vi "shag_start — 8.vi"() -> ()   [LabVIEW 2016]
uses:
  <vilib>/Instr/_visa.llb/VISA Configure Serial Port (Instr).vi
panel:
  out "text":string
  out "2":i32
  out "1":i32
  out "text2":string
  out "положение в мин 2":i32
  out "положение в мин 1":i32
  in  "all":T1(tab)
  out "положение шд 2":i32(knob) scale=-10.0..190.0
  out "текущее положение 2":string
  out "положение в минутах 2":string
  in  "Минуты 2":i32 min=-600 max=11400
  in  "Stop двигатель 2":bool
  in  "Вращение по градусам +  2":bool
  in  "Вращение по градусам -  2":bool
  in  "Вернуться в нулевое положение 2":bool
  in  "Задать текущее положение нулевым 2":bool
  in  "Установка минут 2":bool
  in  "Блокировать трубку №2":bool
  out "положение шд":i32(knob) scale=-10.0..190.0
  out "текущее положение":string
  out "положение в минутах 1":string
  in  "Минуты":i32 min=-600 max=11400
  in  "Stop двигатель":bool
  in  "Вращение по градусам +":bool
  in  "Вращение по градусам -":bool
  in  "Вернуться в нулевое положение":bool
  in  "Задать текущее положение нулевым":bool
  in  "Установка минут":bool
  in  "Блокировать зеркало №1":bool
  in  "stop":bool
  in  "Выберете COM порт":refnum<visa-resource-name>="COM1"
  in  "Скорость обмена данными":u32(ring)=19200 items=["9600"=9600, "19200"=19200, "38400"=38400, "57600"=57600]
  in  "Число бит на символ":u16=8 min=5 max=8 step=1
  in  "Контроль чётности":enum16{"None", "Odd", "Even", "Mark", "Space"}(ring)
  in  "Стоповый бит":u16(ring)=10 items=["1.0"=10, "1.5"=15, "2.0"=20]
  in  "Контроль переполнения":u16(ring) items=["None"=0, "XON/XOFF"=1, "RTS/CTS"=2, "DTR/DSR"=4]
  # "1 - адресс 1 двигателя\n2 - адресс 2 двигателя\n$0MV\\01+   - запуск всех двигателей в положительном направлении \n$0MS\\00   - остановка всех двигателей\n$0MJ\\04+\\00\\00\\01   - 1 шаг всех двигателей\n$0SS\\01\\10   - скорость 10 для всех двигателей"
  # "Поворотный стол"
  # "Ренгеновская трубка №2"
  # "Положение:"
  # "Зеркало №1"
  # "Положение:"
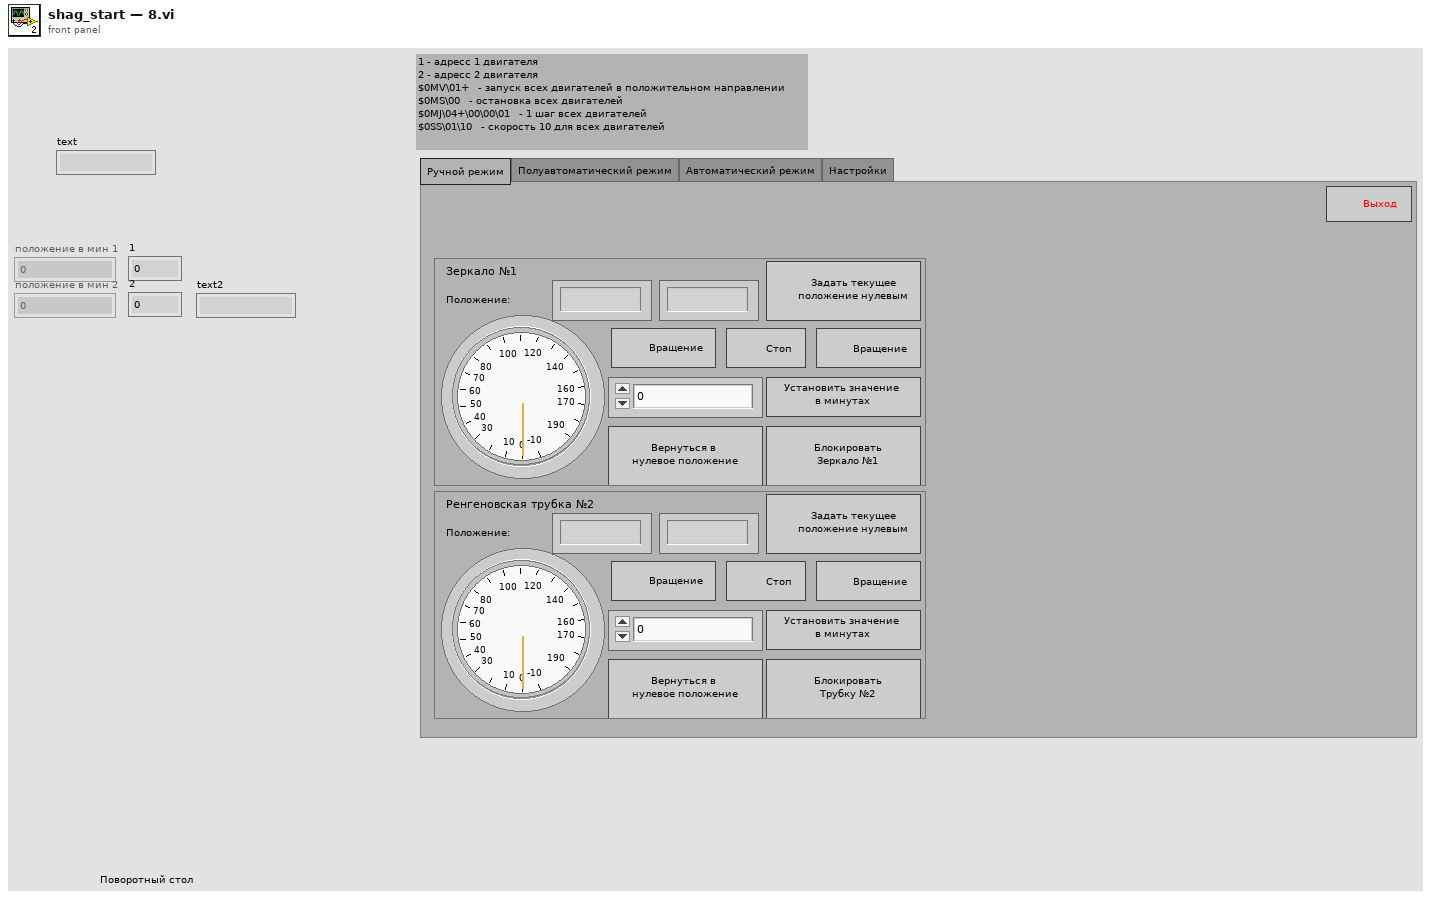
[diagram p1: front panel]
types:
  T1 = enum32{"Ручной режим", "Полуавтоматический режим", "Автоматический режим", "Настройки"}
  T2 = enum16{"open", "replace", "create", "open or create", "replace or create", "replace or create with confirmation"}
  T3 = enum8{"Enabled", "Disabled", "Disabled and Grayed Out"}
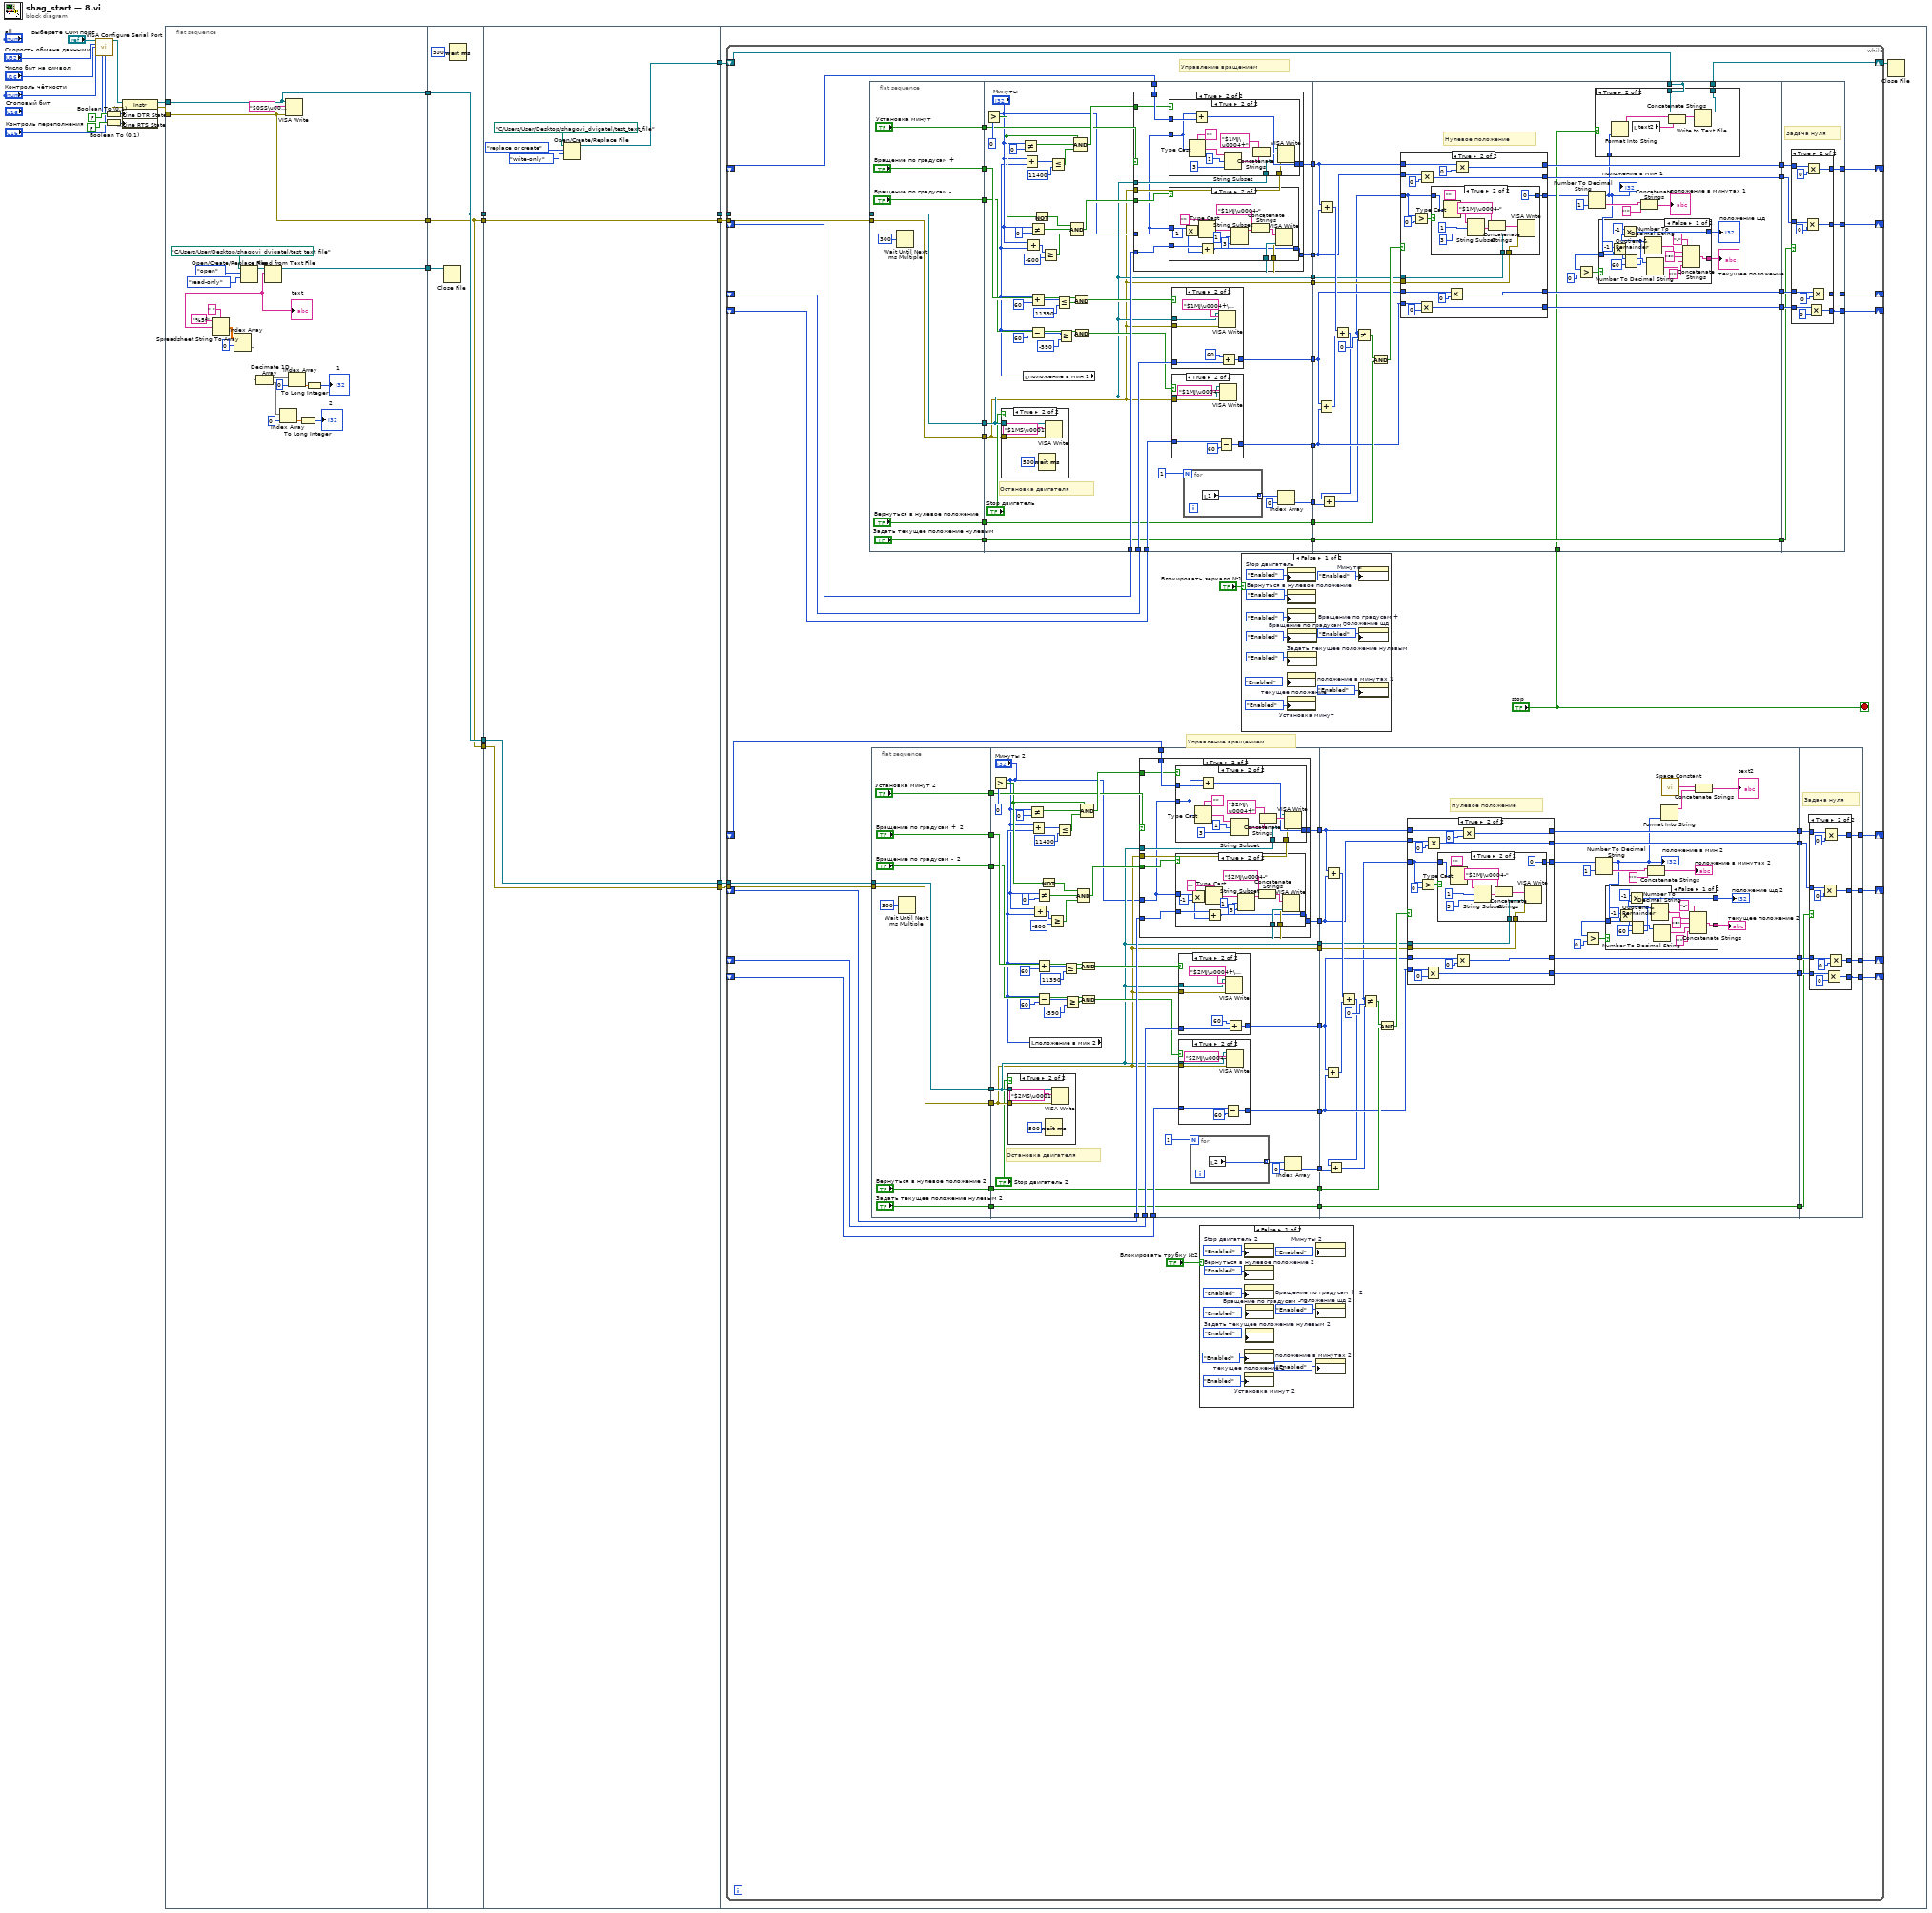
[diagram p0: block diagram]
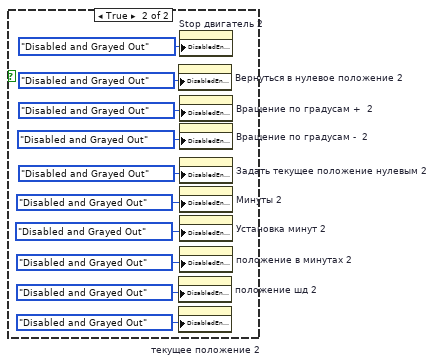
[diagram p2: hidden frame]
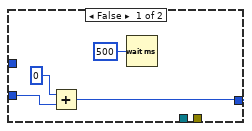
[diagram p4: hidden frame]
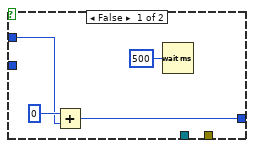
[diagram p5: hidden frame]
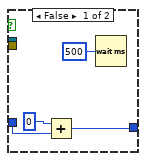
[diagram p7: hidden frame]
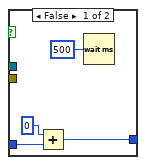
[diagram p8: hidden frame]
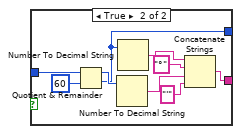
[diagram p9: hidden frame]
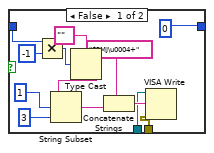
[diagram p11: hidden frame]
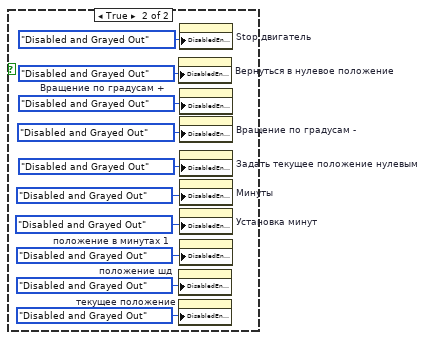
[diagram p13: hidden frame]
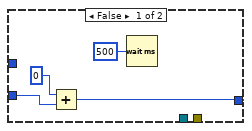
[diagram p15: hidden frame]
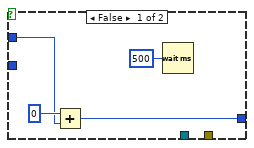
[diagram p16: hidden frame]
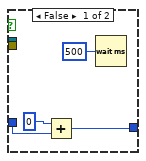
[diagram p18: hidden frame]
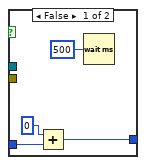
[diagram p19: hidden frame]
diagram:
  n1 = call-poly "VISA Configure Serial Port"("VISA resource name"="Выберете COM порт", "baud rate (9600)"="Скорость обмена данными", "data bits (8)"="Число бит на символ", "parity (0:none)"="Контроль чётности", "stop bits (10: 1 bit)"="Стоповый бит", "flow control (0:none)"="Контроль переполнения") -> ("VISA resource name out"=w24:refnum<visa-resource-name>, "error out"=w23:errorcluster)  [unwired: 8 in]
  n2 = Boolean To (0,1)(Boolean=FALSE ("DTR Write")) -> (0, 1=w25:i16)
  n3 = Boolean To (0,1)(Boolean=FALSE ("DTR Write")) -> (0, 1=w26:i16)
  n4 = property class="Instr"(reference=w24, error in=w23, "Serial Settings:Modem Line Settings:Line DTR State"=w25, "Serial Settings:Modem Line Settings:Line RTS State"=w26) -> (reference out=w22:refnum<visa-resource-name>, error out=w21:errorcluster)
  n5 = flat-sequence {
    tunnel: w22 -> [w47]
    tunnel: w21 -> [w46]
    tunnel: [w47] -> w20
    tunnel: [w46] -> w19
    tunnel: [w42] -> w10
    tunnel: [w51] -> w9
    tunnel: w20 -> [w51]
    tunnel: w19 -> [w50]
    tunnel: [w50] -> w7
    tunnel: [w51] -> w5
    tunnel: [w50] -> w3
    tunnel: w10 -> [w49]
    tunnel: w9 -> [w60]
    tunnel: [w60] -> w8
    tunnel: w7 -> [w59]
    tunnel: [w59] -> w6
    tunnel: w5 -> [w58]
    tunnel: [w58] -> w4
    tunnel: w3 -> [w57]
    tunnel: [w57] -> w2
    tunnel: [w53] -> w1
    tunnel: w8 -> [w66]
    tunnel: w6 -> [w65]
    tunnel: w4 -> [w61]
    tunnel: w2 -> [w64]
    tunnel: w1 -> [w63]
    frame #0 {
      n6 = Open/Create/Replace File(file path (use dialog)=path "C:/Users/User/Desktop/shagovi_dvigatel/test_text_file", operation (0:open)=T2."open", access (0:read/write)=enum16{"read/write", "read-only", "write-only"}."read-only") -> (refnum out=w41:refnum<file>)  [unwired: 3 in, 2 out]
      n7 = Read from Text File(file (use dialog)=w41) -> (refnum out=w42:refnum<file>, text=w27:string)  [unwired: 3 in, 2 out]
      "text" <- w27
      n8 = Spreadsheet String To Array(delimiter (Tab)=" ", format string="%5f", spreadsheet string=w27) -> (array=w38:dbl[][])  [unwired: 1 in]
      n9 = Index Array(array=w38, index (row)=0 ("index")) -> (element=w36:dbl[])  [unwired: 1 in]
      n10 = Decimate 1D Array(w36) -> (w32:dbl[], w34:dbl[])
      n11 = Index Array(array=w34, index=0) -> (element=w31:dbl)
      n12 = VISA Write(VISA resource name=w47, write buffer="$0SS\u0001\u0010", error in (no error)=w46) -> ()  [unwired: 3 out]
      n13 = Index Array(array=w32, index=0) -> (element=w30:dbl)
      n14 = To Long Integer(number=w31) -> (32bit integer=→"2":i32)
      n15 = To Long Integer(number=w30) -> (32bit integer=→"1":i32)
    }
    frame #1 {
      n16 = Close File(refnum=w49) -> ()  [unwired: 1 in, 2 out]
      n17 = Wait (ms)(milliseconds to wait=u32 500) -> ()  [unwired: 1 out]
    }
    frame #2 {
      n18 = Open/Create/Replace File(file path (use dialog)=path "C:/Users/User/Desktop/shagovi_dvigatel/test_text_file", operation (0:open)=T2."replace or create", access (0:read/write)=enum16{"read/write", "read-only", "write-only"}."write-only") -> (refnum out=w53:refnum<file>)  [unwired: 3 in, 2 out]
    }
    frame #3 {
      n19 = while {
        tunnel: w66 -> [w109]
        tunnel: w65 -> [w108]
        shift-right: [w104] -> _
        shift-left: _ -> [w113]
        shift-right: [w105] -> _
        shift-left: _ -> [w112]
        shift-right: [w106] -> _
        shift-left: _ -> [w111]
        shift-right: [w107] -> _
        shift-left: _ -> [w110]
        tunnel: w64 -> [w78]
        shift-right: [w100] -> w62
        shift-left: w63 -> [w101]
        tunnel: w61 -> [w77]
        shift-right: [w73] -> _
        shift-left: _ -> [w74]
        shift-right: [w71] -> _
        shift-left: _ -> [w72]
        shift-right: [w69] -> _
        shift-left: _ -> [w70]
        shift-right: [w67] -> _
        shift-left: _ -> [w68]
        stop <- "stop" stop-if-true
        # "Управление вращением"
        # "Управление вращением"
        n20 = flat-sequence {
          tunnel: w108 -> [w432]
          tunnel: w109 -> [w433]
          tunnel: [w433] -> w133
          tunnel: [w432] -> w132
          tunnel: ["Вращение по градусам +"] -> w131
          tunnel: ["Вращение по градусам -"] -> w130
          tunnel: ["Вернуться в нулевое положение"] -> w129
          tunnel: ["Задать текущее положение нулевым"] -> w128
          tunnel: ["Установка минут"] -> w127
          tunnel: w133 -> [w457]
          tunnel: w132 -> [w439]
          tunnel: [w480] -> w126
          tunnel: w113 -> [w477]
          tunnel: w112 -> [w479]
          tunnel: [w478] -> w125
          tunnel: w111 -> [w476]
          tunnel: w110 -> [w475]
          tunnel: w131 -> [w461]
          tunnel: w130 -> [w460]
          tunnel: [w474] -> w124
          tunnel: [w473] -> w123
          tunnel: [w458] -> w122
          tunnel: w129 -> [w458]
          tunnel: [w439] -> w121
          tunnel: [w457] -> w120
          tunnel: [w456] -> w119
          tunnel: w128 -> [w456]
          tunnel: w127 -> [w450]
          tunnel: [w437] -> w102
          tunnel: w126 -> [w562]
          tunnel: w125 -> [w563]
          tunnel: [w582] -> w118
          tunnel: [w580] -> w117
          tunnel: w124 -> [w564]
          tunnel: w123 -> [w565]
          tunnel: [w571] -> w116
          tunnel: [w578] -> w115
          tunnel: w122 -> [w574]
          tunnel: w121 -> [w570]
          tunnel: w120 -> [w569]
          tunnel: w119 -> [w567]
          tunnel: [w567] -> w114
          tunnel: [w556] -> _
          tunnel: "stop" -> [w559]
          tunnel: w101 -> [w556]
          tunnel: w102 -> [w551]
          tunnel: [w552] -> w100
          tunnel: [w668] -> w104
          tunnel: [w665] -> w105
          tunnel: w118 -> [w667]
          tunnel: w117 -> [w666]
          tunnel: [w664] -> w106
          tunnel: [w663] -> w107
          tunnel: w116 -> [w662]
          tunnel: w115 -> [w661]
          tunnel: w114 -> [w660]
          frame #0 {
            n21 = Wait Until Next ms Multiple(millisecond multiple=u32 300) -> ()  [unwired: 1 out]
          }
          frame #1 {
            # "Остановка двигателя"
            n22 = Greater?(x="Минуты", y=0) -> (0:w448:bool)
            n23 = case shown="True" "Stop двигатель" {
              tunnel: w457 -> [_ w528]
              tunnel: w439 -> [_ w527]
              frame False {
              }
              frame True {
                n24 = Wait (ms)(milliseconds to wait=u32 500) -> ()  [unwired: 1 out]
                n25 = VISA Write(VISA resource name=w528, write buffer="$1MS\u0001", error in (no error)=w527) -> ()  [unwired: 3 out]
              }
            }
            n26 = Not Equal?(x="Минуты", y=0) -> (x != y?=w447:bool)
            n27 = local read "положение в мин 1"() -> (w438:i32)
            n28 = Add(x="Минуты", y=w438) -> (x+y=w471:i32)
            n29 = Add(x="Минуты", y=w438) -> (x+y=w442:i32)
            n30 = Not Equal?(x="Минуты", y=0) -> (x != y?=w445:bool)
            n31 = Add(x=w438, y=60) -> (x+y=w466:i32)
            n32 = Subtract(x=w438, y=60) -> (x-y=w453:i32)
            n33 = Not(x=w448) -> (.not. x?=w449:bool)
            n34 = Greater Or Equal?(x=w442, y=-600) -> (x >= y?=w443:bool)
            n35 = Less Or Equal?(x=w471, y=11400) -> (x <= y?=w446:bool)
            n36 = Less Or Equal?(x=w466, y=11390) -> (x <= y?=w463:bool)
            n37 = Greater Or Equal?(x=w453, y=-590) -> (x >= y?=w454:bool)
            n38 = Compound Arithmetic op=AND(w449, w445, w443) -> (w467:bool)
            n39 = And(x=w461, y=w463) -> (x .and. y?=w462:bool)
            n40 = And(x=w460, y=w454) -> (x .and. y?=w459:bool)
            n41 = Compound Arithmetic op=AND(w448, w447, w446) -> (w469:bool)
            n42 = case shown="True" w450 {
              tunnel: [w483 w492] -> w480
              tunnel: w479 -> [w482 w491]
              tunnel: [w482 w490] -> w478
              tunnel: w477 -> [w483 w489]
              tunnel: w469 -> [_ w488]
              tunnel: w467 -> [_ w487]
              tunnel: w439 -> [_ w486]
              tunnel: w457 -> [_ w485]
              tunnel: "Минуты" -> [_ w484]
              frame False {
              }
              frame True {
                n43 = case shown="True" w488 {
                  tunnel: [w513 w519] -> w492
                  tunnel: w489 -> [w512 w518]
                  tunnel: w486 -> [_ w517]
                  tunnel: w485 -> [_ w516]
                  tunnel: w484 -> [_ w515]
                  frame False {
                    n44 = Add(x=0, y=w512) -> (x+y=w513:i32)
                    n45 = Wait (ms)(milliseconds to wait=u32 500) -> ()  [unwired: 1 out]
                  }
                  frame True {
                    n46 = Type Cast(type="", x=w515) -> (*(type *) &x=w522:string)
                    n47 = Add(x=w515, y=w518) -> (x+y=w519:i32)
                    n48 = String Subset(string=w522, offset (0)=1, length (rest)=3 ("length (rest)")) -> (substring=w521:string)
                    n49 = Concatenate Strings("$1MJ\u0004+" ("write buffer"), w521) -> (w525:string)
                    n50 = VISA Write(VISA resource name=w516, write buffer=w525, error in (no error)=w517) -> ()  [unwired: 3 out]
                  }
                }
                n51 = case shown="True" w487 {
                  tunnel: [w495 w501] -> w490
                  tunnel: w491 -> [w494 w500]
                  tunnel: w485 -> [_ w503]
                  tunnel: w486 -> [_ w502]
                  tunnel: w484 -> [_ w497]
                  frame False {
                    n52 = Add(x=0, y=w494) -> (x+y=w495:i32)
                    n53 = Wait (ms)(milliseconds to wait=u32 500) -> ()  [unwired: 1 out]
                  }
                  frame True {
                    n54 = Multiply(x=w497, y=-1) -> (x*y=w499:i32)
                    n55 = Type Cast(type="", x=w499) -> (*(type *) &x=w506:string)
                    n56 = Add(x=w500, y=w497) -> (x+y=w501:i32)
                    n57 = String Subset(string=w506, offset (0)=1, length (rest)=3 ("length (rest)")) -> (substring=w505:string)
                    n58 = Concatenate Strings("$1MJ\u0004-" ("write buffer"), w505) -> (w509:string)
                    n59 = VISA Write(VISA resource name=w503, write buffer=w509, error in (no error)=w502) -> ()  [unwired: 3 out]
                  }
                }
              }
            }
            n60 = case shown="True" w462 {
              tunnel: [w543 w550] -> w474
              tunnel: w476 -> [w542 w545]
              tunnel: w457 -> [_ w546]
              tunnel: w439 -> [_ w547]
              frame False {
                n61 = Add(x=0, y=w542) -> (x+y=w543:i32)
                n62 = Wait (ms)(milliseconds to wait=u32 500) -> ()  [unwired: 1 out]
              }
              frame True {
                n63 = VISA Write(VISA resource name=w546, write buffer="$1MJ\u0004+\u0000\u0000<", error in (no error)=w547) -> ()  [unwired: 3 out]
                n64 = Add(x=60, y=w545) -> (x+y=w550:i32)
              }
            }
            n65 = case shown="True" w459 {
              tunnel: [w533 w536] -> w473
              tunnel: w475 -> [w532 w535]
              tunnel: w457 -> [_ w539]
              tunnel: w439 -> [_ w538]
              frame False {
                n66 = Add(x=0, y=w532) -> (x+y=w533:i32)
                n67 = Wait (ms)(milliseconds to wait=u32 500) -> ()  [unwired: 1 out]
              }
              frame True {
                n68 = Subtract(x=w535, y=60 ("x")) -> (x-y=w536:i32)
                n69 = VISA Write(VISA resource name=w539, write buffer="$1MJ\u0004-\u0000\u0000<", error in (no error)=w538) -> ()  [unwired: 3 out]
              }
            }
            n70 = for {
              N: 1 -> [_]
              tunnel: [w481] -> w435 mode=indexing
              n71 = local read "1"() -> (w481:i32)
            }
            n72 = Index Array(array=w435, index=0) -> (element=w437:i32)
          }
          frame #2 {
            # "Нулевое положение"
            n73 = Add(x=w564, y=w565) -> (x+y=w575:i32)
            n74 = Add(x=w562, y=w563) -> (x+y=w579:i32)
            n75 = Add(x=w579, y=w575) -> (x+y=w554:i32)
            n76 = Add(x=w554, y=w551) -> (x+y=w553:i32)
            n77 = Not Equal?(x=w553, y=0 ("x")) -> (x != y?=w572:bool)
            n78 = And(x=w572, y=w574) -> (x .and. y?=w581:bool)
            n79 = case shown="True" w581 {
              tunnel: [w613 w635] -> w555
              tunnel: w562 -> [w617 w632]
              tunnel: [w617 w631] -> w582
              tunnel: [w616 w630] -> w580
              tunnel: w553 -> [w613 w624]
              tunnel: [w614 w626] -> w578
              tunnel: [w615 w623] -> w571
              tunnel: w563 -> [w616 w622]
              tunnel: w570 -> [_ w621]
              tunnel: w569 -> [_ w620]
              tunnel: w564 -> [w615 w619]
              tunnel: w565 -> [w614 w618]
              frame False {
              }
              frame True {
                n80 = Greater?(x=w624, y=0) -> (0:w625:bool)
                n81 = Multiply(x=w618, y=0) -> (x*y=w626:i32)
                n82 = Multiply(x=w622, y=0) -> (x*y=w630:i32)
                n83 = case shown="True" w625 {
                  tunnel: w624 -> [w640 w653]
                  tunnel: [0 0] -> w635
                  tunnel: w620 -> [w637 w650]
                  tunnel: w621 -> [w636 w649]
                  frame False {
                    n84 = Multiply(x=w640, y=-1) -> (x*y=w638:i32)
                    n85 = Type Cast(type="", x=w638) -> (*(type *) &x=w644:string)
                    n86 = String Subset(string=w644, offset (0)=1, length (rest)=3 ("length (rest)")) -> (substring=w643:string)
                    n87 = Concatenate Strings("$1MJ\u0004+" ("write buffer"), w643) -> (w647:string)
                    n88 = VISA Write(VISA resource name=w637, write buffer=w647, error in (no error)=w636) -> ()  [unwired: 3 out]
                  }
                  frame True {
                    n89 = Type Cast(type="", x=w653) -> (*(type *) &x=w656:string)
                    n90 = String Subset(string=w656, offset (0)=1, length (rest)=3 ("length (rest)")) -> (substring=w655:string)
                    n91 = Concatenate Strings("$1MJ\u0004-" ("write buffer"), w655) -> (w651:string)
                    n92 = VISA Write(VISA resource name=w650, write buffer=w651, error in (no error)=w649) -> ()  [unwired: 3 out]
                  }
                }
                n93 = Multiply(x=w619, y=0) -> (x*y=w623:i32)
                n94 = Multiply(x=w632, y=0) -> (x*y=w631:i32)
              }
            }
            "положение в мин 1" <- w555
            n95 = Greater?(x=w555, y=0) -> (0:w577:bool)
            n96 = Number To Decimal String(number=w555, width (-)=i16 1) -> (decimal integer string=w558:string)
            n97 = case shown="True" w559 {
              tunnel: w556 -> [w583 w588]
              tunnel: w555 -> [_ w589]
              tunnel: [w583 w587] -> w552
              frame False {
              }
              frame True {
                n98 = Format Into String(w589) -> (resulting string=w585:string)  [unwired: 3 in, 1 out]
                n99 = local read "text2"() -> (w584:string)
                n100 = Concatenate Strings(w585, w584) -> (w586:string)
                n101 = Write to Text File(file (use dialog)=w588, text=w586) -> (refnum out=w587:refnum<file>)  [unwired: 2 in, 2 out]
              }
            }
            n102 = case shown="False" w577 {
              tunnel: w555 -> [w596 w612]
              tunnel: [w600 w606] -> w568
              tunnel: [w590 w604] -> w566
              frame False {
                n103 = Multiply(x=-1, y=w596) -> (x*y=w595:i32)
                n104 = Quotient & Remainder(x=w595, y=60) -> (x-y*floor(x/y)=w599:i32, floor(x/y)=w591:i32)
                n105 = Multiply(x=-1, y=w591) -> (x*y=w590:i32)
                n106 = Number To Decimal String(number=w591) -> (decimal integer string=w597:string)  [unwired: 1 in]
                n107 = Number To Decimal String(number=w599) -> (decimal integer string=w598:string)  [unwired: 1 in]
                n108 = Concatenate Strings("-" ("string"), w597, "°" ("string"), w598, "'" ("string")) -> (w600:string)
              }
              frame True {
                n109 = Quotient & Remainder(x=w612, y=60) -> (x-y*floor(x/y)=w605:i32, floor(x/y)=w604:i32)
                n110 = Number To Decimal String(number=w605) -> (decimal integer string=w607:string)  [unwired: 1 in]
                n111 = Number To Decimal String(number=w604) -> (decimal integer string=w608:string)  [unwired: 1 in]
                n112 = Concatenate Strings(w608, "°" ("string"), w607, "'" ("string")) -> (w606:string)
              }
            }
            "положение шд" <- w566
            "текущее положение" <- w568
            n113 = Concatenate Strings(w558, "'" ("string")) -> (→"положение в минутах 1":string)
          }
          frame #3 {
            # "Задача нуля"
            n114 = case shown="True" w660 {
              tunnel: [w672 w683] -> w668
              tunnel: w667 -> [w672 w684]
              tunnel: w666 -> [w671 w680]
              tunnel: [w671 w679] -> w665
              tunnel: [w670 w676] -> w664
              tunnel: [w669 w675] -> w663
              tunnel: w662 -> [w670 w674]
              tunnel: w661 -> [w669 w673]
              frame False {
              }
              frame True {
                n115 = Multiply(x=w680, y=0) -> (x*y=w679:i32)
                n116 = Multiply(x=w684, y=0) -> (x*y=w683:i32)
                n117 = Multiply(x=w673, y=0) -> (x*y=w675:i32)
                n118 = Multiply(x=w674, y=0) -> (x*y=w676:i32)
              }
            }
          }
        }
        n119 = flat-sequence {
          tunnel: w78 -> [w160]
          tunnel: w77 -> [w161]
          tunnel: [w161] -> w99
          tunnel: [w160] -> w98
          tunnel: ["Вращение по градусам +  2"] -> w97
          tunnel: ["Вращение по градусам -  2"] -> w96
          tunnel: ["Вернуться в нулевое положение 2"] -> w95
          tunnel: ["Задать текущее положение нулевым 2"] -> w94
          tunnel: ["Установка минут 2"] -> w93
          tunnel: w99 -> [w185]
          tunnel: w98 -> [w169]
          tunnel: [w208] -> w92
          tunnel: w74 -> [w205]
          tunnel: w72 -> [w207]
          tunnel: [w206] -> w91
          tunnel: w70 -> [w204]
          tunnel: w68 -> [w203]
          tunnel: w97 -> [w189]
          tunnel: w96 -> [w188]
          tunnel: [w202] -> w90
          tunnel: [w201] -> w89
          tunnel: [w186] -> w88
          tunnel: w95 -> [w186]
          tunnel: [w169] -> w87
          tunnel: [w185] -> w86
          tunnel: [w184] -> w85
          tunnel: w94 -> [w184]
          tunnel: w93 -> [w178]
          tunnel: [w167] -> w84
          tunnel: w92 -> [w292]
          tunnel: w91 -> [w293]
          tunnel: [w310] -> w83
          tunnel: [w308] -> w82
          tunnel: w90 -> [w294]
          tunnel: w89 -> [w295]
          tunnel: [w299] -> w81
          tunnel: [w306] -> w80
          tunnel: w88 -> [w302]
          tunnel: w87 -> [w298]
          tunnel: w86 -> [w297]
          tunnel: w85 -> [w296]
          tunnel: [w296] -> w79
          tunnel: w84 -> [w279]
          tunnel: [w389] -> w73
          tunnel: [w386] -> w71
          tunnel: w83 -> [w388]
          tunnel: w82 -> [w387]
          tunnel: [w385] -> w69
          tunnel: [w384] -> w67
          tunnel: w81 -> [w383]
          tunnel: w80 -> [w382]
          tunnel: w79 -> [w381]
          frame #0 {
            n120 = Wait Until Next ms Multiple(millisecond multiple=u32 300) -> ()  [unwired: 1 out]
          }
          frame #1 {
            # "Остановка двигателя"
            n121 = Greater?(x="Минуты 2", y=0) -> (0:w176:bool)
            n122 = case shown="True" "Stop двигатель 2" {
              tunnel: w185 -> [_ w256]
              tunnel: w169 -> [_ w255]
              frame False {
              }
              frame True {
                n123 = Wait (ms)(milliseconds to wait=u32 500) -> ()  [unwired: 1 out]
                n124 = VISA Write(VISA resource name=w256, write buffer="$2MS\u0001", error in (no error)=w255) -> ()  [unwired: 3 out]
              }
            }
            n125 = Not Equal?(x="Минуты 2", y=0) -> (x != y?=w175:bool)
            n126 = local read "положение в мин 2"() -> (w168:i32)
            n127 = Add(x="Минуты 2", y=w168) -> (x+y=w199:i32)
            n128 = Add(x="Минуты 2", y=w168) -> (x+y=w171:i32)
            n129 = Not Equal?(x="Минуты 2", y=0) -> (x != y?=w173:bool)
            n130 = Add(x=w168, y=60) -> (x+y=w194:i32)
            n131 = Subtract(x=w168, y=60) -> (x-y=w181:i32)
            n132 = Not(x=w176) -> (.not. x?=w177:bool)
            n133 = Greater Or Equal?(x=w171, y=-600) -> (x >= y?=w172:bool)
            n134 = Less Or Equal?(x=w199, y=11400) -> (x <= y?=w174:bool)
            n135 = Less Or Equal?(x=w194, y=11390) -> (x <= y?=w191:bool)
            n136 = Greater Or Equal?(x=w181, y=-590) -> (x >= y?=w182:bool)
            n137 = Compound Arithmetic op=AND(w177, w173, w172) -> (w195:bool)
            n138 = And(x=w189, y=w191) -> (x .and. y?=w190:bool)
            n139 = And(x=w188, y=w182) -> (x .and. y?=w187:bool)
            n140 = Compound Arithmetic op=AND(w176, w175, w174) -> (w197:bool)
            n141 = case shown="True" w178 {
              tunnel: [w211 w220] -> w208
              tunnel: w207 -> [w210 w219]
              tunnel: [w210 w218] -> w206
              tunnel: w205 -> [w211 w217]
              tunnel: w197 -> [_ w216]
              tunnel: w195 -> [_ w215]
              tunnel: w169 -> [_ w214]
              tunnel: w185 -> [_ w213]
              tunnel: "Минуты 2" -> [_ w212]
              frame False {
              }
              frame True {
                n142 = case shown="True" w216 {
                  tunnel: [w241 w247] -> w220
                  tunnel: w217 -> [w240 w246]
                  tunnel: w214 -> [_ w245]
                  tunnel: w213 -> [_ w244]
                  tunnel: w212 -> [_ w243]
                  frame False {
                    n143 = Add(x=0, y=w240) -> (x+y=w241:i32)
                    n144 = Wait (ms)(milliseconds to wait=u32 500) -> ()  [unwired: 1 out]
                  }
                  frame True {
                    n145 = Type Cast(type="", x=w243) -> (*(type *) &x=w250:string)
                    n146 = Add(x=w243, y=w246) -> (x+y=w247:i32)
                    n147 = String Subset(string=w250, offset (0)=1, length (rest)=3 ("length (rest)")) -> (substring=w249:string)
                    n148 = Concatenate Strings("$2MJ\u0004+" ("write buffer"), w249) -> (w253:string)
                    n149 = VISA Write(VISA resource name=w244, write buffer=w253, error in (no error)=w245) -> ()  [unwired: 3 out]
                  }
                }
                n150 = case shown="True" w215 {
                  tunnel: [w223 w229] -> w218
                  tunnel: w219 -> [w222 w228]
                  tunnel: w213 -> [_ w231]
                  tunnel: w214 -> [_ w230]
                  tunnel: w212 -> [_ w225]
                  frame False {
                    n151 = Add(x=0, y=w222) -> (x+y=w223:i32)
                    n152 = Wait (ms)(milliseconds to wait=u32 500) -> ()  [unwired: 1 out]
                  }
                  frame True {
                    n153 = Multiply(x=w225, y=-1) -> (x*y=w227:i32)
                    n154 = Type Cast(type="", x=w227) -> (*(type *) &x=w234:string)
                    n155 = Add(x=w228, y=w225) -> (x+y=w229:i32)
                    n156 = String Subset(string=w234, offset (0)=1, length (rest)=3 ("length (rest)")) -> (substring=w233:string)
                    n157 = Concatenate Strings("$2MJ\u0004-" ("write buffer"), w233) -> (w237:string)
                    n158 = VISA Write(VISA resource name=w231, write buffer=w237, error in (no error)=w230) -> ()  [unwired: 3 out]
                  }
                }
              }
            }
            n159 = case shown="True" w190 {
              tunnel: [w271 w278] -> w202
              tunnel: w204 -> [w270 w273]
              tunnel: w185 -> [_ w274]
              tunnel: w169 -> [_ w275]
              frame False {
                n160 = Add(x=0, y=w270) -> (x+y=w271:i32)
                n161 = Wait (ms)(milliseconds to wait=u32 500) -> ()  [unwired: 1 out]
              }
              frame True {
                n162 = VISA Write(VISA resource name=w274, write buffer="$2MJ\u0004+\u0000\u0000<", error in (no error)=w275) -> ()  [unwired: 3 out]
                n163 = Add(x=60, y=w273) -> (x+y=w278:i32)
              }
            }
            n164 = case shown="True" w187 {
              tunnel: [w261 w264] -> w201
              tunnel: w203 -> [w260 w263]
              tunnel: w185 -> [_ w267]
              tunnel: w169 -> [_ w266]
              frame False {
                n165 = Add(x=0, y=w260) -> (x+y=w261:i32)
                n166 = Wait (ms)(milliseconds to wait=u32 500) -> ()  [unwired: 1 out]
              }
              frame True {
                n167 = Subtract(x=w263, y=60 ("x")) -> (x-y=w264:i32)
                n168 = VISA Write(VISA resource name=w267, write buffer="$2MJ\u0004-\u0000\u0000<", error in (no error)=w266) -> ()  [unwired: 3 out]
              }
            }
            n169 = for {
              N: 1 -> [_]
              tunnel: [w209] -> w165 mode=indexing
              n170 = local read "2"() -> (w209:i32)
            }
            n171 = Index Array(array=w165, index=0) -> (element=w167:i32)
          }
          frame #2 {
            # "Нулевое положение"
            n172 = Add(x=w294, y=w295) -> (x+y=w303:i32)
            n173 = Add(x=w292, y=w293) -> (x+y=w307:i32)
            n174 = Add(x=w307, y=w303) -> (x+y=w288:i32)
            n175 = Add(x=w288, y=w279) -> (x+y=w287:i32)
            n176 = Not Equal?(x=w287, y=0 ("x")) -> (x != y?=w300:bool)
            n177 = And(x=w300, y=w302) -> (x .and. y?=w309:bool)
            n178 = case shown="True" w309 {
              tunnel: [w334 w356] -> w281
              tunnel: w292 -> [w338 w353]
              tunnel: [w338 w352] -> w310
              tunnel: [w337 w351] -> w308
              tunnel: w287 -> [w334 w345]
              tunnel: [w335 w347] -> w306
              tunnel: [w336 w344] -> w299
              tunnel: w293 -> [w337 w343]
              tunnel: w298 -> [_ w342]
              tunnel: w297 -> [_ w341]
              tunnel: w294 -> [w336 w340]
              tunnel: w295 -> [w335 w339]
              frame False {
              }
              frame True {
                n179 = Greater?(x=w345, y=0) -> (0:w346:bool)
                n180 = Multiply(x=w339, y=0) -> (x*y=w347:i32)
                n181 = Multiply(x=w343, y=0) -> (x*y=w351:i32)
                n182 = case shown="True" w346 {
                  tunnel: w345 -> [w361 w374]
                  tunnel: [0 0] -> w356
                  tunnel: w341 -> [w358 w371]
                  tunnel: w342 -> [w357 w370]
                  frame False {
                    n183 = Multiply(x=w361, y=-1) -> (x*y=w359:i32)
                    n184 = Type Cast(type="", x=w359) -> (*(type *) &x=w365:string)
                    n185 = String Subset(string=w365, offset (0)=1, length (rest)=3 ("length (rest)")) -> (substring=w364:string)
                    n186 = Concatenate Strings("$2MJ\u0004+" ("write buffer"), w364) -> (w368:string)
                    n187 = VISA Write(VISA resource name=w358, write buffer=w368, error in (no error)=w357) -> ()  [unwired: 3 out]
                  }
                  frame True {
                    n188 = Type Cast(type="", x=w374) -> (*(type *) &x=w377:string)
                    n189 = String Subset(string=w377, offset (0)=1, length (rest)=3 ("length (rest)")) -> (substring=w376:string)
                    n190 = Concatenate Strings("$2MJ\u0004-" ("write buffer"), w376) -> (w372:string)
                    n191 = VISA Write(VISA resource name=w371, write buffer=w372, error in (no error)=w370) -> ()  [unwired: 3 out]
                  }
                }
                n192 = Multiply(x=w340, y=0) -> (x*y=w344:i32)
                n193 = Multiply(x=w353, y=0) -> (x*y=w352:i32)
              }
            }
            "положение в мин 2" <- w281
            n194 = Greater?(x=w281, y=0) -> (0:w305:bool)
            n195 = Number To Decimal String(number=w281, width (-)=i16 1) -> (decimal integer string=w290:string)
            n196 = case shown="False" w305 {
              tunnel: w281 -> [w317 w333]
              tunnel: [w321 w327] -> w285
              tunnel: [w311 w325] -> w284
              frame False {
                n197 = Multiply(x=-1, y=w317) -> (x*y=w316:i32)
                n198 = Quotient & Remainder(x=w316, y=60) -> (x-y*floor(x/y)=w320:i32, floor(x/y)=w312:i32)
                n199 = Multiply(x=-1, y=w312) -> (x*y=w311:i32)
                n200 = Number To Decimal String(number=w312) -> (decimal integer string=w318:string)  [unwired: 1 in]
                n201 = Number To Decimal String(number=w320) -> (decimal integer string=w319:string)  [unwired: 1 in]
                n202 = Concatenate Strings("-" ("string"), w318, "°" ("string"), w319, "'" ("string")) -> (w321:string)
              }
              frame True {
                n203 = Quotient & Remainder(x=w333, y=60) -> (x-y*floor(x/y)=w326:i32, floor(x/y)=w325:i32)
                n204 = Number To Decimal String(number=w326) -> (decimal integer string=w328:string)  [unwired: 1 in]
                n205 = Number To Decimal String(number=w325) -> (decimal integer string=w329:string)  [unwired: 1 in]
                n206 = Concatenate Strings(w329, "°" ("string"), w328, "'" ("string")) -> (w327:string)
              }
            }
            "положение шд 2" <- w284
            "текущее положение 2" <- w285
            n207 = Concatenate Strings(w290, "'" ("string")) -> (→"положение в минутах 2":string)
            n208 = Format Into String(w281) -> (resulting string=w282:string)  [unwired: 3 in, 1 out]
            n209 = call <vilib>:"Space Constant.vi"() -> ("String"=w280:string)
            n210 = Concatenate Strings(w280, w282) -> (→"text2":string)
          }
          frame #3 {
            # "Задача нуля"
            n211 = case shown="True" w381 {
              tunnel: [w393 w404] -> w389
              tunnel: w388 -> [w393 w405]
              tunnel: w387 -> [w392 w401]
              tunnel: [w392 w400] -> w386
              tunnel: [w391 w397] -> w385
              tunnel: [w390 w396] -> w384
              tunnel: w383 -> [w391 w395]
              tunnel: w382 -> [w390 w394]
              frame False {
              }
              frame True {
                n212 = Multiply(x=w401, y=0) -> (x*y=w400:i32)
                n213 = Multiply(x=w405, y=0) -> (x*y=w404:i32)
                n214 = Multiply(x=w394, y=0) -> (x*y=w396:i32)
                n215 = Multiply(x=w395, y=0) -> (x*y=w397:i32)
              }
            }
          }
        }
        n216 = case shown="False" "Блокировать трубку №2" {
          frame False {
            n217 = property on="Stop двигатель 2" class="Bool"("DisabledEnum"=T3."Enabled" ("Disabled")) -> ()  [unwired: 2 in, 2 out]
            n218 = property on="Вернуться в нулевое положение 2" class="Bool"("DisabledEnum"=T3."Enabled" ("Disabled")) -> ()  [unwired: 2 in, 2 out]
            n219 = property on="Вращение по градусам +  2" class="Bool"("DisabledEnum"=T3."Enabled" ("Disabled")) -> ()  [unwired: 2 in, 2 out]
            n220 = property on="текущее положение 2" class="Str"("DisabledEnum"=T3."Enabled" ("Disabled")) -> ()  [unwired: 2 in, 2 out]
            n221 = property on="Установка минут 2" class="Bool"("DisabledEnum"=T3."Enabled" ("Disabled")) -> ()  [unwired: 2 in, 2 out]
            n222 = property on="Вращение по градусам -  2" class="Bool"("DisabledEnum"=T3."Enabled" ("Disabled")) -> ()  [unwired: 2 in, 2 out]
            n223 = property on="Задать текущее положение нулевым 2" class="Bool"("DisabledEnum"=T3."Enabled" ("Disabled")) -> ()  [unwired: 2 in, 2 out]
            n224 = property on="Минуты 2" class="DigNum (strict)"("DisabledEnum"=T3."Enabled" ("Disabled")) -> ()  [unwired: 2 in, 2 out]
            n225 = property on="положение шд 2" class="Knob (strict)"("DisabledEnum"=T3."Enabled" ("Disabled")) -> ()  [unwired: 2 in, 2 out]
            n226 = property on="положение в минутах 2" class="Str"("DisabledEnum"=T3."Enabled" ("Disabled")) -> ()  [unwired: 2 in, 2 out]
          }
          frame True {
            n227 = property on="Вернуться в нулевое положение 2" class="Bool"("DisabledEnum"=T3."Disabled and Grayed Out" ("Disabled")) -> ()  [unwired: 2 in, 2 out]
            n228 = property on="положение шд 2" class="Knob (strict)"("DisabledEnum"=T3."Disabled and Grayed Out" ("Disabled")) -> ()  [unwired: 2 in, 2 out]
            n229 = property on="текущее положение 2" class="Str"("DisabledEnum"=T3."Disabled and Grayed Out" ("Disabled")) -> ()  [unwired: 2 in, 2 out]
            n230 = property on="Stop двигатель 2" class="Bool"("DisabledEnum"=T3."Disabled and Grayed Out" ("Disabled")) -> ()  [unwired: 2 in, 2 out]
            n231 = property on="Вращение по градусам +  2" class="Bool"("DisabledEnum"=T3."Disabled and Grayed Out" ("Disabled")) -> ()  [unwired: 2 in, 2 out]
            n232 = property on="Вращение по градусам -  2" class="Bool"("DisabledEnum"=T3."Disabled and Grayed Out" ("Disabled")) -> ()  [unwired: 2 in, 2 out]
            n233 = property on="Задать текущее положение нулевым 2" class="Bool"("DisabledEnum"=T3."Disabled and Grayed Out" ("Disabled")) -> ()  [unwired: 2 in, 2 out]
            n234 = property on="Минуты 2" class="DigNum (strict)"("DisabledEnum"=T3."Disabled and Grayed Out" ("Disabled")) -> ()  [unwired: 2 in, 2 out]
            n235 = property on="Установка минут 2" class="Bool"("DisabledEnum"=T3."Disabled and Grayed Out" ("Disabled")) -> ()  [unwired: 2 in, 2 out]
            n236 = property on="положение в минутах 2" class="Str"("DisabledEnum"=T3."Disabled and Grayed Out" ("Disabled")) -> ()  [unwired: 2 in, 2 out]
          }
        }
        n237 = case shown="False" "Блокировать зеркало №1" {
          frame False {
            n238 = property on="Stop двигатель" class="Bool"("DisabledEnum"=T3."Enabled" ("Disabled")) -> ()  [unwired: 2 in, 2 out]
            n239 = property on="Вернуться в нулевое положение" class="Bool"("DisabledEnum"=T3."Enabled" ("Disabled")) -> ()  [unwired: 2 in, 2 out]
            n240 = property on="Вращение по градусам +" class="Bool"("DisabledEnum"=T3."Enabled" ("Disabled")) -> ()  [unwired: 2 in, 2 out]
            n241 = property on="текущее положение" class="Str"("DisabledEnum"=T3."Enabled" ("Disabled")) -> ()  [unwired: 2 in, 2 out]
            n242 = property on="Установка минут" class="Bool"("DisabledEnum"=T3."Enabled" ("Disabled")) -> ()  [unwired: 2 in, 2 out]
            n243 = property on="Вращение по градусам -" class="Bool"("DisabledEnum"=T3."Enabled" ("Disabled")) -> ()  [unwired: 2 in, 2 out]
            n244 = property on="Задать текущее положение нулевым" class="Bool"("DisabledEnum"=T3."Enabled" ("Disabled")) -> ()  [unwired: 2 in, 2 out]
            n245 = property on="Минуты" class="DigNum (strict)"("DisabledEnum"=T3."Enabled" ("Disabled")) -> ()  [unwired: 2 in, 2 out]
            n246 = property on="положение шд" class="Knob (strict)"("DisabledEnum"=T3."Enabled" ("Disabled")) -> ()  [unwired: 2 in, 2 out]
            n247 = property on="положение в минутах 1" class="Str"("DisabledEnum"=T3."Enabled" ("Disabled")) -> ()  [unwired: 2 in, 2 out]
          }
          frame True {
            n248 = property on="Вернуться в нулевое положение" class="Bool"("DisabledEnum"=T3."Disabled and Grayed Out" ("Disabled")) -> ()  [unwired: 2 in, 2 out]
            n249 = property on="положение шд" class="Knob (strict)"("DisabledEnum"=T3."Disabled and Grayed Out" ("Disabled")) -> ()  [unwired: 2 in, 2 out]
            n250 = property on="текущее положение" class="Str"("DisabledEnum"=T3."Disabled and Grayed Out" ("Disabled")) -> ()  [unwired: 2 in, 2 out]
            n251 = property on="Stop двигатель" class="Bool"("DisabledEnum"=T3."Disabled and Grayed Out" ("Disabled")) -> ()  [unwired: 2 in, 2 out]
            n252 = property on="Вращение по градусам +" class="Bool"("DisabledEnum"=T3."Disabled and Grayed Out" ("Disabled")) -> ()  [unwired: 2 in, 2 out]
            n253 = property on="Вращение по градусам -" class="Bool"("DisabledEnum"=T3."Disabled and Grayed Out" ("Disabled")) -> ()  [unwired: 2 in, 2 out]
            n254 = property on="Задать текущее положение нулевым" class="Bool"("DisabledEnum"=T3."Disabled and Grayed Out" ("Disabled")) -> ()  [unwired: 2 in, 2 out]
            n255 = property on="Минуты" class="DigNum (strict)"("DisabledEnum"=T3."Disabled and Grayed Out" ("Disabled")) -> ()  [unwired: 2 in, 2 out]
            n256 = property on="Установка минут" class="Bool"("DisabledEnum"=T3."Disabled and Grayed Out" ("Disabled")) -> ()  [unwired: 2 in, 2 out]
            n257 = property on="положение в минутах 1" class="Str"("DisabledEnum"=T3."Disabled and Grayed Out" ("Disabled")) -> ()  [unwired: 2 in, 2 out]
          }
        }
      }
      n258 = Close File(refnum=w62) -> ()  [unwired: 1 in, 2 out]
    }
  }
